vi "PerfAddRemove.vi"() -> (3 "Add mean":dbl format="%.2p")   [LabVIEW 2024, in "TypedCircularBuffer.Tests.Perf.lvlib"]
uses:
  TypedCircularBuffer.Tests.Perf.lvlib
  TypedCircularBuffer.lvclass/TypedCircularBuffer.ctl
  Type.ctl
  IsFull.vi
  TypedCircularBuffer.lvclass
  <vilib>/Analysis/NI_AALBase.lvlib
panel:
  out "Add standard deviation":dbl format="%.2p"
  out "Remove standard deviation":dbl format="%.2p"
  out "Remove mean":dbl format="%.2p"
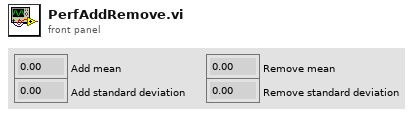
[diagram p1: front panel]
types:
  T1 = typedef "TypedCircularBuffer.lvclass/Type.ctl" = i32
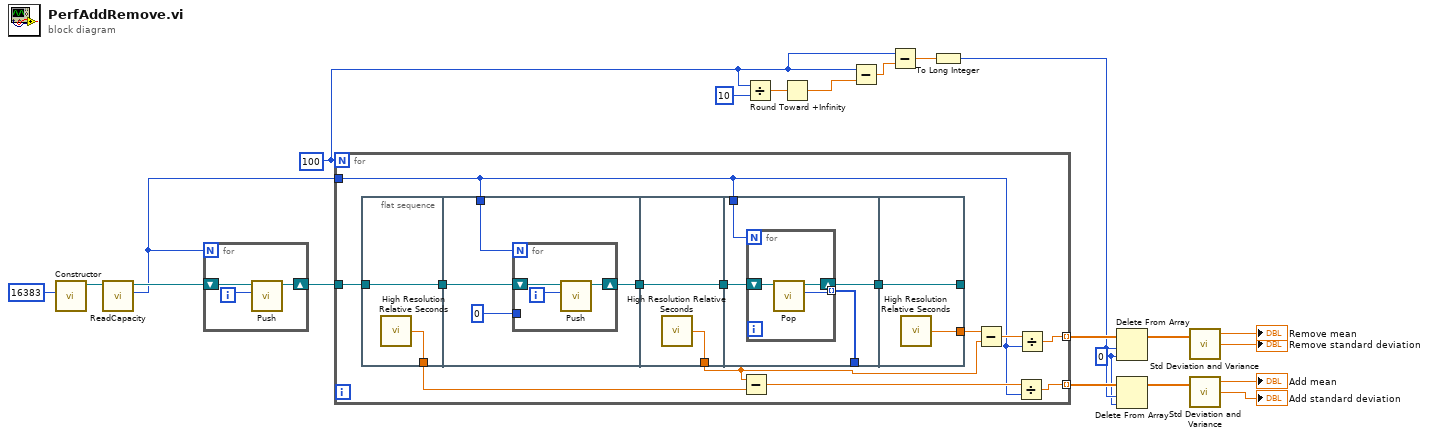
[diagram p0: block diagram]
diagram:
  w5 = 0 ("index")
  w10 = 100
  n1 = call "Constructor.vi"("Capacity"=u32 16383) -> ("TypedCircularBuffer out"=w16:refnum<class "TypedCircularBuffer.lvclass">)  [unwired: 10 in]
  n2 = call "ReadCapacity.vi"("TypedCircularBuffer in"=w16) -> ("capacity"=w1:u32, "TypedCircularBuffer out"=w3:refnum<class "TypedCircularBuffer.lvclass">)  [unwired: 9 in]
  n3 = for {
    N: w1 -> [_]
    shift-right: [w23] -> w2
    shift-left: w3 -> [w24]
    i -> [w22]
    n4 = call "Push.vi"("Element"=w22, "TypedCircularBuffer in"=w24) -> ("TypedCircularBuffer out"=w23:refnum<class "TypedCircularBuffer.lvclass">)  [unwired: 7 in, 2 out]
  }
  n5 = for {
    N: w10 -> [_]
    tunnel: [w27] -> w9 mode=indexing
    tunnel: w2 -> [w36]
    tunnel: [w28] -> w8 mode=indexing
    tunnel: w1 -> [w25]
    n6 = flat-sequence {
      tunnel: w36 -> [w39]
      tunnel: [w39] -> w33
      tunnel: [w38] -> w31
      tunnel: [w42] -> w34
      tunnel: w33 -> [w43]
      tunnel: w25 -> [w40]
      tunnel: [w48] -> w32
      tunnel: [w47] -> w35
      tunnel: w34 -> [w47]
      tunnel: w35 -> [w52]
      tunnel: [w51] -> _
      tunnel: w25 -> [w50]
      tunnel: [w49] -> w26
      tunnel: [w57] -> w37
      tunnel: [w56] -> _
      tunnel: w26 -> [w56]
      frame #0 {
        n7 = call <vilib>:"High Resolution Relative Seconds.vi"() -> ("relative seconds"=w38:dbl)
      }
      frame #1 {
        n8 = for {
          N: w40 -> [_]
          shift-right: [w45] -> w42
          shift-left: w43 -> [w46]
          tunnel: T1 0 ("Element") -> [_]
          i -> [w44]
          n9 = call "Push.vi"("Element"=w44, "TypedCircularBuffer in"=w46) -> ("TypedCircularBuffer out"=w45:refnum<class "TypedCircularBuffer.lvclass">)  [unwired: 7 in, 2 out]
        }
      }
      frame #2 {
        n10 = call <vilib>:"High Resolution Relative Seconds.vi"() -> ("relative seconds"=w48:dbl)
      }
      frame #3 {
        n11 = for {
          N: w50 -> [_]
          shift-right: [w54] -> w49
          shift-left: w52 -> [w55]
          tunnel: [w53] -> w51 mode=indexing
          n12 = call "Pop.vi"("TypedCircularBuffer in"=w55) -> ("element"=w53:T1, "TypedCircularBuffer out"=w54:refnum<class "TypedCircularBuffer.lvclass">)  [unwired: 8 in, 1 out]
        }
      }
      frame #4 {
        n13 = call <vilib>:"High Resolution Relative Seconds.vi"() -> ("relative seconds"=w57:dbl)
      }
    }
    n14 = Subtract(x=w32, y=w31) -> (x-y=w29:dbl)
    n15 = Subtract(x=w37, y=w32) -> (x-y=w30:dbl)
    n16 = Divide(x=w29, y=w25) -> (x/y=w28:dbl)
    n17 = Divide(x=w30, y=w25) -> (x/y=w27:dbl)
  }
  n18 = Divide(x=w10, y=10) -> (x/y=w14:dbl)
  n19 = Round Toward +Infinity(x=w14) -> (ceil(x): smallest int >= x=w13:dbl)
  n20 = Subtract(x=w10, y=w13) -> (x-y=w12:dbl)
  n21 = Subtract(x=w10, y=w12) -> (x-y=w11:dbl)
  n22 = To Long Integer(number=w11) -> (32bit integer=w6:i32)
  n23 = Delete From Array(array=w9, length=w6, index=w5) -> (array with subset deleted=w4:dbl[])  [unwired: 1 out]
  n24 = Delete From Array(array=w8, length=w6, index=w5) -> (array with subset deleted=w7:dbl[])  [unwired: 1 out]
  n25 = call <vilib>:"Std Deviation and Variance.vi"("X"=w4) -> ("mean"=→"Remove mean":dbl, "standard deviation"=→"Remove standard deviation":dbl)  [unwired: 1 in, 1 out]
  n26 = call <vilib>:"Std Deviation and Variance.vi"("X"=w7) -> ("mean"=→"Add mean":dbl, "standard deviation"=→"Add standard deviation":dbl)  [unwired: 1 in, 1 out]
